vi "Configure Gamepad.vi"(6 "Cluster 2":T2, 7 "invert z":refnum<vi>, 8 "Slide 3":cluster{u32, u32, u32}(slide)={7, 6, 2} scale=0.0..7.0, 9 "invert y":refnum<vi>, 10 "invert x":refnum<vi>, 11 "device ID":refnum<k1>) -> (0 "Slide-Function":cluster{u32, u32, u32}(slide)={5, 2, 0} scale=0.0..7.0, 1 "Slide Raw":cluster{u32, u32, u32}(slide)={5, 2, 0} scale=0.0..7.0)   [LabVIEW 2012]
uses:
  <vilib>/Utility/miscctls.llb/LVPointTypeDef.ctl
  <vilib>/Utility/inputDevices.llb/joystickAcquire.vi
panel:
  out "Settings Refrences 2":T1
  in  "Invert":bool=TRUE
  in  "closed?":bool
  in  "Invert":bool
  in  "Invert":bool=TRUE
  in  "xr":u16(ring)=1 items=["1 X"=1, "2 A"=2, "3 B"=3, "4 Y"=4, "5 LB"=5, "6 RB"=6, "7 LT"=7, "8 RT"=8, "9 Back"=9]
  in  "yf":u16(ring)=4 items=["1 X"=1, "2 A"=2, "3 B"=3, "4 Y"=4, "5 LB"=5, "6 RB"=6, "7 LT"=7, "8 RT"=8, "9 Back"=9]
  in  "yr":u16(ring)=2 items=["1 X"=1, "2 A"=2, "3 B"=3, "4 Y"=4, "5 LB"=5, "6 RB"=6, "7 LT"=7, "8 RT"=8, "9 Back"=9]
  in  "xf":u16(ring)=3 items=["1 X"=1, "2 A"=2, "3 B"=3, "4 Y"=4, "5 LB"=5, "6 RB"=6, "7 LT"=7, "8 RT"=8, "9 Back"=9]
  in  "zb":u16(ring)=8 items=["1 X"=1, "2 A"=2, "3 B"=3, "4 Y"=4, "5 LB"=5, "6 RB"=6, "7 LT"=7, "8 RT"=8, "9 Back"=9]
  in  "zf":u16(ring)=6 items=["1 X"=1, "2 A"=2, "3 B"=3, "4 Y"=4, "5 LB"=5, "6 RB"=6, "7 LT"=7, "8 RT"=8, "9 Back"=9]
  in  "halt 2":u16(ring)=9 items=["1 X"=1, "2 A"=2, "3 B"=3, "4 Y"=4, "5 LB"=5, "6 RB"=6, "7 LT"=7, "8 RT"=8, "9 Back"=9]
  out "Joystick Readings":T3
  # "Drag the M1 (green), M2 (red), and M3 (blue) axis pointers to the indicators for the Gamepad Joysticks desired for Microdrive control. \n\nToggle the desired joystick on the gamepad and watch \"Joystick Readings\" to find the correct indicator.\n\nIf you are toggling the left  joystick or D-pad and none of the readings change, press the mode button on your game pad, then try again."
  # "Close window when finished re-configuring gamepad"
  # "Gamepad Mapping\nof Single Step Buttons"
  # "Click on the text in one of the squares and a list of button options will apear. Select the desired gamepad button from the list."
  # "M1"
  # "M2 Axis"
  # "M3"
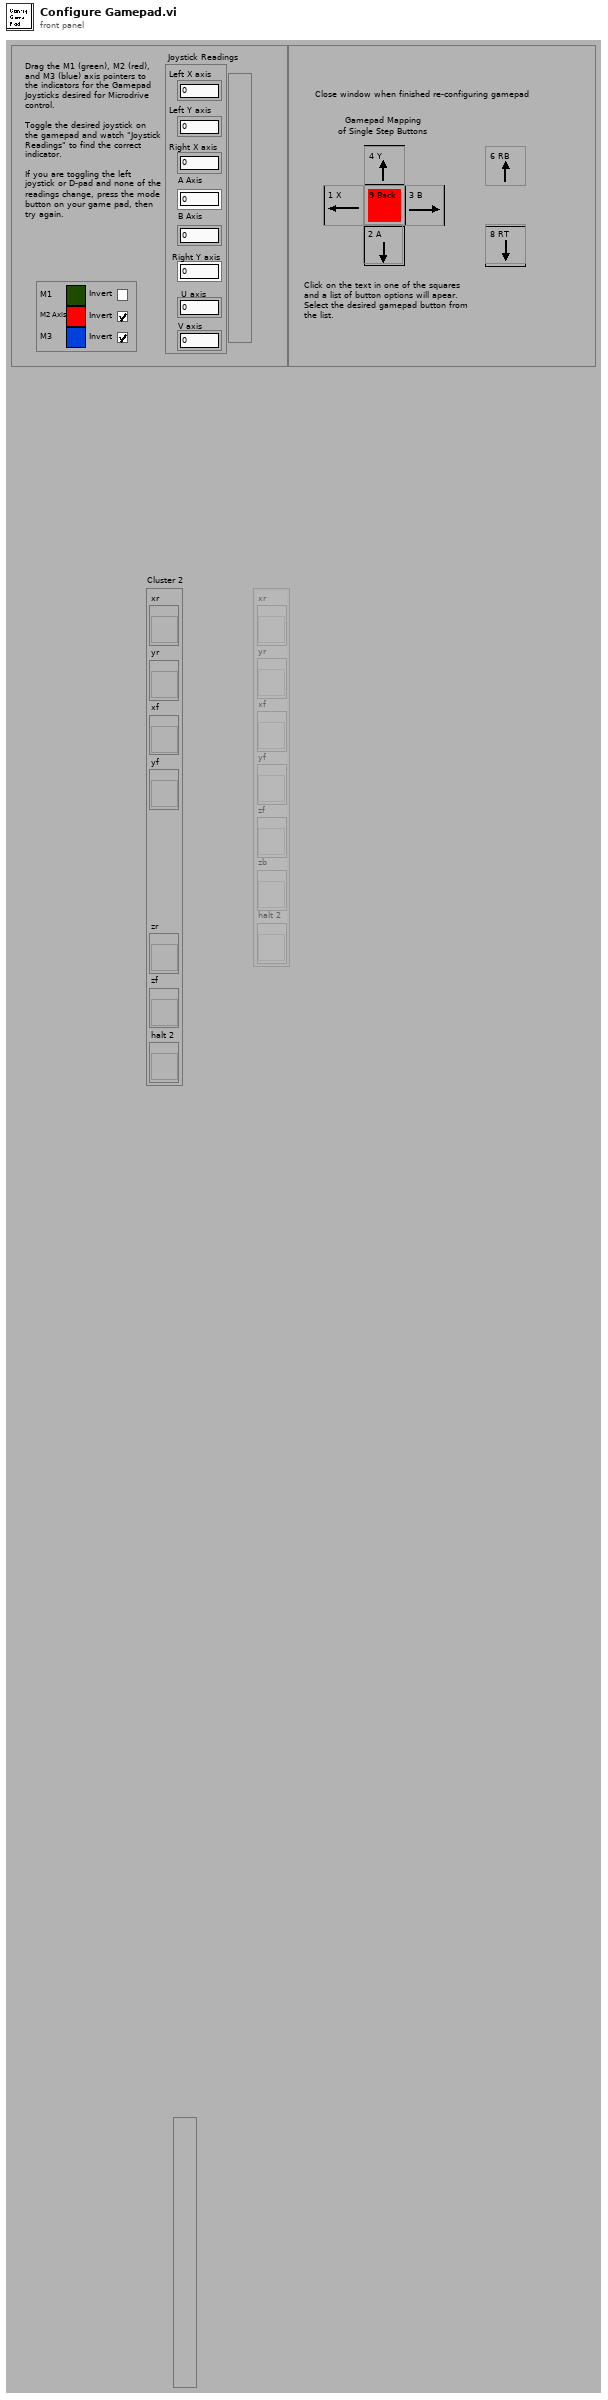
[diagram p1: front panel]
types:
  T1 = cluster{"xr":refnum<vi>, "yr":refnum<vi>, "xf":refnum<vi>, "yf":refnum<vi>, "zb":refnum<vi>, "zf":refnum<vi>, "halt 2":refnum<vi>}
  T2 = cluster{"xr":refnum<vi>, "yr":refnum<vi>, "xf":refnum<vi>, "yf":refnum<vi>, "zr":refnum<vi>, "zf":refnum<vi>, "halt 2":refnum<vi>}
  T3 = cluster{"Left X axis":i32, "Left Y axis":i32, "Right X axis":i32, "A Axis":i32, "B Axis":i32, "Right Y axis":i32, "U axis":i32, "V axis":i32}
  T4 = typedef "LVPointTypeDef.ctl" = cluster{"Horizontal":i16, "Vertical":i16}
  T5 = cluster{"X axis":i32, "Y axis":i32, "Z axis":i32, "X axis rotation":i32, "Y axis rotation":i32, "Z axis rotation":i32, "U axis":i32, "V axis":i32}
  T6 = cluster{"Right X axis":i32, "Right Y axis":i32, "Left X axis":i32, "A Axis":i32, "B Axis":i32, "Left Y axis":i32, "U axis":i32, "V axis":i32}
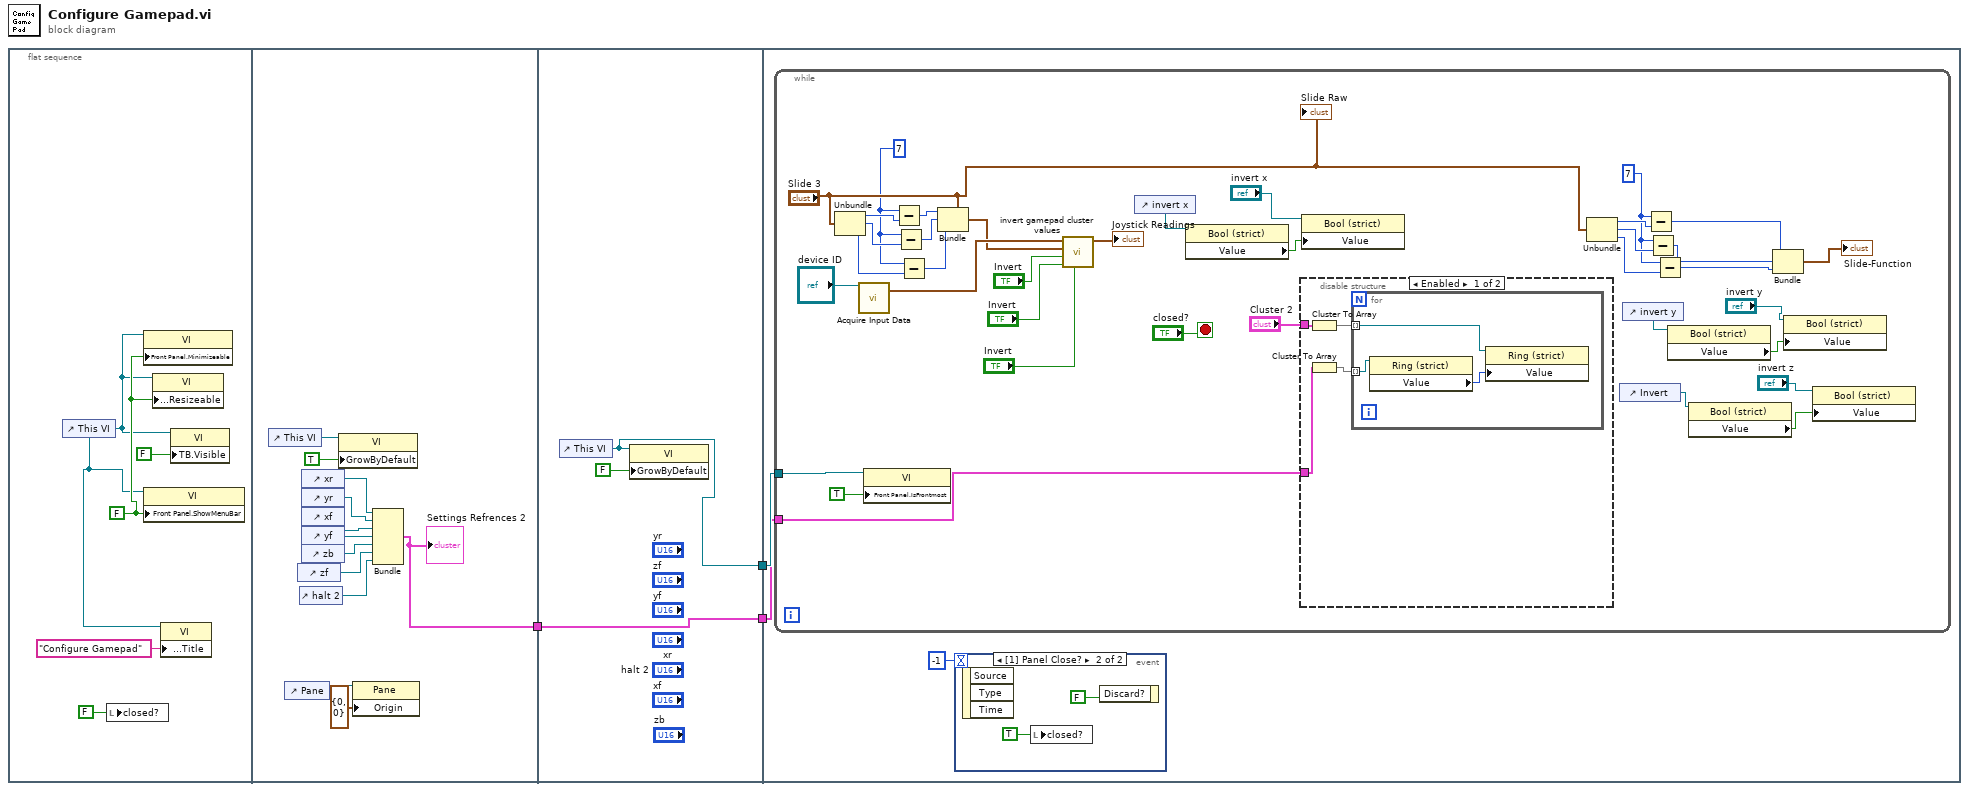
[diagram p0: block diagram]
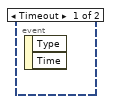
[diagram p2: hidden frame]
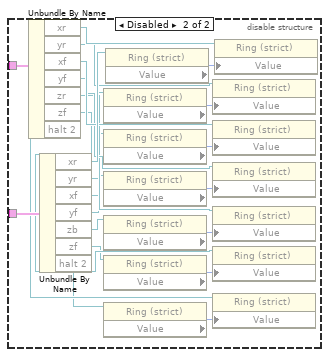
[diagram p3: hidden frame]
diagram:
  n1 = flat-sequence {
    tunnel: [w9] -> w1
    tunnel: [w22] -> w3
    tunnel: [w21] -> w2
    tunnel: w1 -> [w21]
    tunnel: w3 -> [w25]
    tunnel: w2 -> [w24]
    frame #0 {
      w5 = FALSE ("Front Panel Window:Show Menu Bar")
      n2 = control-ref of="This VI"() -> (w4:refnum<vi>)
      n3 = local write "closed?"(FALSE ("closed?")) -> ()
      n4 = property class="VI"(reference=w4, "Front Panel.Minimizeable"=w5) -> ()  [unwired: 1 in, 2 out]
      n5 = property class="VI"(reference=w4, "Front Panel.ShowMenuBar"=w5) -> ()  [unwired: 1 in, 2 out]
      n6 = property class="VI"(reference=w4, "Front Panel.Resizeable"=w5) -> ()  [unwired: 1 in, 2 out]
      n7 = property class="VI"(reference=w4, "Front Panel.Title"="Configure Gamepad" ("Front Panel Window:Title")) -> ()  [unwired: 1 in, 2 out]
      n8 = property class="VI"(reference=w4, "TB.Visible"=FALSE ("Tool Bar:Visible")) -> ()  [unwired: 1 in, 2 out]
    }
    frame #1 {
      n9 = control-ref of="This VI"() -> (w20:refnum<vi>)
      n10 = control-ref of="Pane"() -> (w14:refnum<vi>)
      n11 = control-ref of="zf"() -> (w10:refnum<vi>)
      n12 = control-ref of="halt 2"() -> (w12:refnum<vi>)
      n13 = control-ref of="xr"() -> (w18:refnum<vi>)
      n14 = control-ref of="yr"() -> (w17:refnum<vi>)
      n15 = control-ref of="xf"() -> (w16:refnum<vi>)
      n16 = control-ref of="yf"() -> (w15:refnum<vi>)
      n17 = control-ref of="zb"() -> (w11:refnum<vi>)
      n18 = property class="VI"(reference=w20, "GrowByDefault"=TRUE ("Expand When Dropped As SubVI")) -> ()  [unwired: 1 in, 2 out]
      n19 = property class="Pane"(reference=w14, "Origin"=T4 {"Horizontal"=0, "Vertical"=0}) -> ()  [unwired: 1 in, 2 out]
      n20 = Bundle("xr"=w18, "yr"=w17, "xf"=w16, "yf"=w15, "zb"=w11, "zf"=w10, "halt 2"=w12) -> (w9:T1)  [unwired: 1 out]
      "Settings Refrences 2" <- w9
    }
    frame #2 {
      n21 = control-ref of="This VI"() -> (w22:refnum<vi>)
      n22 = property class="VI"(reference=w22, "GrowByDefault"=FALSE ("Expand When Dropped As SubVI")) -> ()  [unwired: 1 in, 2 out]
    }
    frame #3 {
      n23 = while {
        tunnel: w25 -> [w45]
        tunnel: w24 -> [w43]
        stop <- "closed?" stop-if-true
        w41 = u32 7 ("x")
        w32 = u32 7 ("x")
        n24 = Unbundle("Slide 3") -> (w60:u32, w59:u32, w31:u32)
        n25 = call-poly <vilib>:"Acquire Input Data.vi"("device ID"="device ID") -> ("axis info"=w64:T5)  [unwired: 1 in, 17 out]
        n26 = property class="VI"(reference=w45, "Front Panel.IsFrontmost"=TRUE ("Front Panel Window:Is Frontmost")) -> ()  [unwired: 1 in, 2 out]
        n27 = Subtract(x=w32, y=w60) -> (x-y=w58:u32)
        n28 = Subtract(x=w32, y=w59) -> (x-y=w57:u32)
        n29 = Subtract(x=w32, y=w31) -> (x-y=w30:u32)
        n30 = Bundle(cluster="Slide 3", w58, w57, w30) -> (w56:cluster{u32, u32, u32})
        n31 = call "invert gamepad cluster values.vi"("Invert Z"="Invert", "Invert Y"="Invert", "Invert X"="Invert", "Slide"=w56, "Joystick Readings"=w64) -> ("Joystick Readings 2"=→"Joystick Readings":T6)  [unwired: 6 out]
        n32 = control-ref of="invert x"() -> (w53:refnum<vi>)
        n33 = property on="Property Node" class="Bool (strict)"(reference=w53) -> ("Value"=w54:bool)  [unwired: 1 in, 2 out]
        n34 = disable-structure shown="Enabled" {
          disable-tunnel: w43 -> [w67 w94]
          disable-tunnel: "Cluster 2" -> [w66 w95]
          frame Enabled {
            n35 = Cluster To Array(cluster=w66) -> (array=w69:refnum<vi>[])
            n36 = Cluster To Array(cluster=w67) -> (array=w68:refnum<vi>[])
            n37 = for {
              tunnel: w69 -> [w70] mode=indexing
              tunnel: w68 -> [w72] mode=indexing
              n38 = property on="Property Node" class="Ring (strict)"(reference=w72) -> ("Value"=w71:u16)  [unwired: 1 in, 2 out]
              n39 = property on="Property Node" class="Ring (strict)"(reference=w70, "Value"=w71) -> ()  [unwired: 1 in, 2 out]
            }
          }
          frame Disabled {
            n40 = Unbundle By Name(w95) -> ("xr"=w92:refnum<vi>, "yr"=w84:refnum<vi>, "xf"=w83:refnum<vi>, "yf"=w82:refnum<vi>, "zr"=w81:refnum<vi>, "zf"=w80:refnum<vi>, "halt 2"=w79:refnum<vi>)
            n41 = Unbundle By Name(w94) -> ("xr"=w93:refnum<vi>, "yr"=w78:refnum<vi>, "xf"=w77:refnum<vi>, "yf"=w76:refnum<vi>, "zb"=w75:refnum<vi>, "zf"=w74:refnum<vi>, "halt 2"=w73:refnum<vi>)
            n42 = property on="Property Node" class="Ring (strict)"(reference=w78) -> ("Value"=w90:u16)  [unwired: 1 in, 2 out]
            n43 = property on="Property Node" class="Ring (strict)"(reference=w77) -> ("Value"=w89:u16)  [unwired: 1 in, 2 out]
            n44 = property on="Property Node" class="Ring (strict)"(reference=w76) -> ("Value"=w88:u16)  [unwired: 1 in, 2 out]
            n45 = property on="Property Node" class="Ring (strict)"(reference=w75) -> ("Value"=w87:u16)  [unwired: 1 in, 2 out]
            n46 = property on="Property Node" class="Ring (strict)"(reference=w74) -> ("Value"=w86:u16)  [unwired: 1 in, 2 out]
            n47 = property on="Property Node" class="Ring (strict)"(reference=w73) -> ("Value"=w85:u16)  [unwired: 1 in, 2 out]
            n48 = property on="Property Node" class="Ring (strict)"(reference=w93) -> ("Value"=w91:u16)  [unwired: 1 in, 2 out]
            n49 = property on="Property Node" class="Ring (strict)"(reference=w84, "Value"=w90) -> ()  [unwired: 1 in, 2 out]
            n50 = property on="Property Node" class="Ring (strict)"(reference=w83, "Value"=w89) -> ()  [unwired: 1 in, 2 out]
            n51 = property on="Property Node" class="Ring (strict)"(reference=w82, "Value"=w88) -> ()  [unwired: 1 in, 2 out]
            n52 = property on="Property Node" class="Ring (strict)"(reference=w81, "Value"=w87) -> ()  [unwired: 1 in, 2 out]
            n53 = property on="Property Node" class="Ring (strict)"(reference=w80, "Value"=w86) -> ()  [unwired: 1 in, 2 out]
            n54 = property on="Property Node" class="Ring (strict)"(reference=w79, "Value"=w85) -> ()  [unwired: 1 in, 2 out]
            n55 = property on="Property Node" class="Ring (strict)"(reference=w92, "Value"=w91) -> ()  [unwired: 1 in, 2 out]
          }
        }
        n56 = property on="Property Node" class="Bool (strict)"(reference="invert x", "Value"=w54) -> ()  [unwired: 1 in, 2 out]
        n57 = Unbundle("Slide 3") -> (w47:u32, w48:u32, w42:u32)
        n58 = control-ref of="Invert"() -> (w35:refnum<vi>)
        n59 = control-ref of="invert y"() -> (w50:refnum<vi>)
        n60 = Subtract(x=w41, y=w47) -> (x-y=w37:u32)
        n61 = Subtract(x=w41, y=w48) -> (x-y=w38:u32)
        n62 = Subtract(x=w41, y=w42) -> (x-y=w39:u32)
        n63 = property on="Property Node" class="Bool (strict)"(reference=w50) -> ("Value"=w51:bool)  [unwired: 1 in, 2 out]
        n64 = property on="Property Node" class="Bool (strict)"(reference=w35) -> ("Value"=w34:bool)  [unwired: 1 in, 2 out]
        n65 = Bundle(w37, w38, w39) -> (→"Slide-Function":cluster{u32, u32, u32})  [unwired: 1 out]
        n66 = property on="Property Node" class="Bool (strict)"(reference="invert y", "Value"=w51) -> ()  [unwired: 1 in, 2 out]
        n67 = property on="Property Node" class="Bool (strict)"(reference="invert z", "Value"=w34) -> ()  [unwired: 1 in, 2 out]
        "Slide Raw" <- "Slide 3"
      }
      n68 = event shown="[1] Panel Close?" {
        selector: _ -> [_ _]
        dyn-events: _ -> [_ _]
        timeout: -1 -> [_ _]
        event Timeout {
          n69 = event-data() -> ()  [unwired: 3 out]
        }
        event Panel Close? {
          n70 = event-data() -> ()  [unwired: 4 out]
          n71 = local write "closed?"(TRUE ("closed?")) -> ()
          n72 = event-data("Discard?"=FALSE) -> ()  [unwired: 1 in, 1 out]
        }
      }
    }
  }
